vi "Climber.vi"() -> ()   [LabVIEW 2012]
uses:
  ClimberState.ctl
  Robot Global Data.vi
  <vilib>/Rock Robotics/WPI/Relay/WPI_RelayValue.ctl
  <vilib>/Rock Robotics/WPI/Solenoid/WPI_SolenoidSetEnum.vi
  <vilib>/Rock Robotics/WPI/Solenoid/WPI_SolenoidValue.ctl
panel:
  in  "Debug":bool
  in  "Step":T1
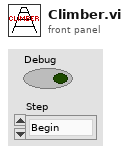
[diagram p1: front panel]
types:
  T1 = typedef "ClimberState.ctl" = enum16{"Begin", "Step 1", "Step 2", "Step 3", "Step 4", "Step 5", "Step 6", "Step 7", "Step 8", "Step 9", "Step 10", "Step 11", "Step 12", "Step 13", "Step 14", "Step 15", "Step 16", "Step 17", "Step 18", "Step 19", "Step 20", "Step 21", "Step 22", "Step 23", "Step 24"}
  T2 = typedef "WPI_RelayValue.ctl" = enum16{"Off", "On", "Forward", "Reverse"}
  T3 = typedef "WPI_SolenoidValue.ctl" = enum16{"Off", "On", "Forward", "Reverse"}
  T4 = typedef "Level state.ctl" = enum16{""}
  T5 = typedef "WPI_RelayDevRef.ctl" = cluster{"DevStatus":errorcluster, "Relay Channel":T6, "Digital Module":T7, "Relay Direction":T8}
  T6 = typedef "FPGA_DIORelayChannel.ctl" = enum8{"Relay 1", "Relay 2", "Relay 3", "Relay 4", "Relay 5", "Relay 6", "Relay 7", "Relay 8", "Invalid"}
  T7 = typedef "FPGA_TypedefDigitalModule.ctl" = enum16{"Digital Module 1", "Digital Module 2"}
  T8 = typedef "WPI_RelayDirection.ctl" = enum16{"Both directions", "Forward only", "Reverse only"}
  T9 = typedef "WPI_MotorControlDeviceRef.ctl" = cluster{"DeviceStatus":errorcluster, "Type":enum16{"PWM", "CAN"}, "PWM":cluster{"Digital Module":T7, "PWM Channel":T10, "DeadBand":T11}, "CAN":cluster{"Device Number":u8, "Control Mode":T12, "Semaphore":T13, "Max Vout":dbl}, "Invert":bool, "TransformRef":T14, "InvTransformRef":T14}
  T10 = typedef "FPGA_DIOPWMChannel.ctl" = enum8{"PWM 1", "PWM 2", "PWM 3", "PWM 4", "PWM 5", "PWM 6", "PWM 7", "PWM 8", "PWM 9", "PWM 10", "Invalid"}
  T11 = typedef "WPI_PWMDeadband.ctl" = cluster{"Name":string, "maxPositivePwm":i32, "minPositivePwm":i32, "centerPwm":i32, "maxNegativePwm":i32, "minNegativePwm":i32, "angularRange":u16}
  T12 = typedef "WPI_CANJaguar_ControlMode.ctl" = enum8{"Percent VBus", "Current", "Speed", "Position", "Voltage"}
  T13 = typedef "Semaphore RefNum" = refnum<k1>
  T14 = typedef "WPI_PWMTransform_ConPane.ctl" = refnum<vi>
  T15 = typedef "WPI_SolenoidDevRef.ctl" = cluster{"DevStatus":errorcluster, "Solenoid Module":T16, "Forward Solenoid Channel":T17, "Reverse Solenoid Channel":T17}
  T16 = typedef "FPGA_TypedefSolenoidModule.ctl" = enum16{"Solenoid Module 1", "Solenoid Module 2"}
  T17 = typedef "WPI_SolenoidChannel.ctl" = enum8{"Solenoid 1", "Solenoid 2", "Solenoid 3", "Solenoid 4", "Solenoid 5", "Solenoid 6", "Solenoid 7", "Solenoid 8", "Invalid"}
  T18 = typedef "WPI_RobotDriveDevRef.ctl" = cluster{"DevStatus":errorcluster, "Motors[]":T9[], "Square Inputs":bool, "Max Output":dbl, "Isochronous":bool}
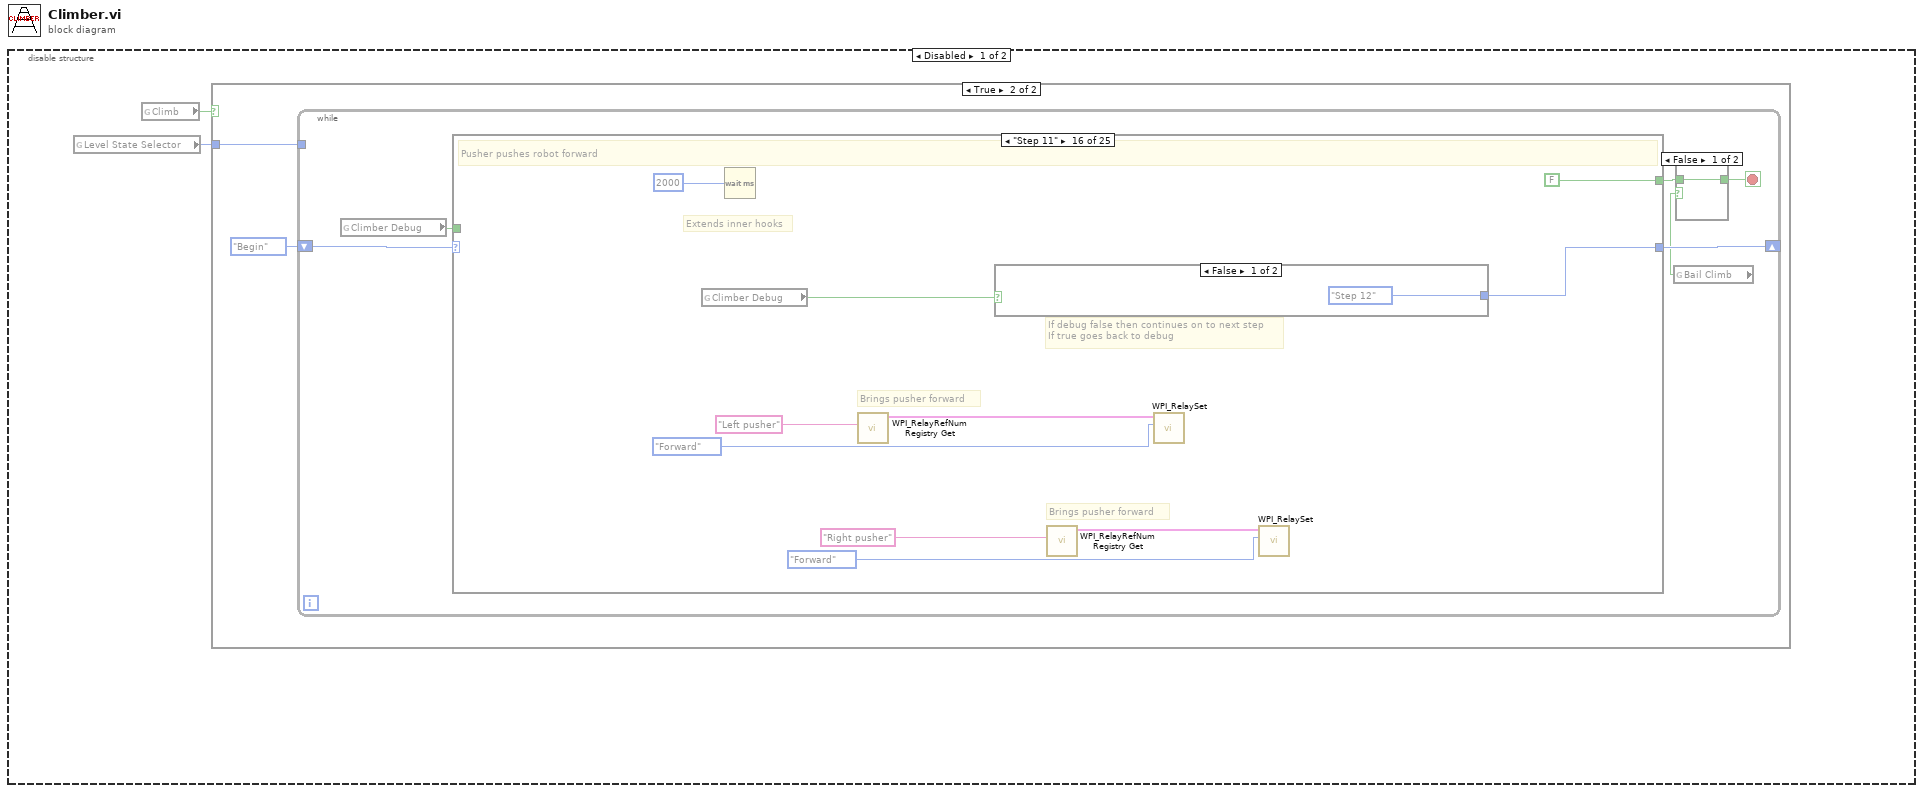
[diagram p0: block diagram]
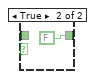
[diagram p3: hidden frame]
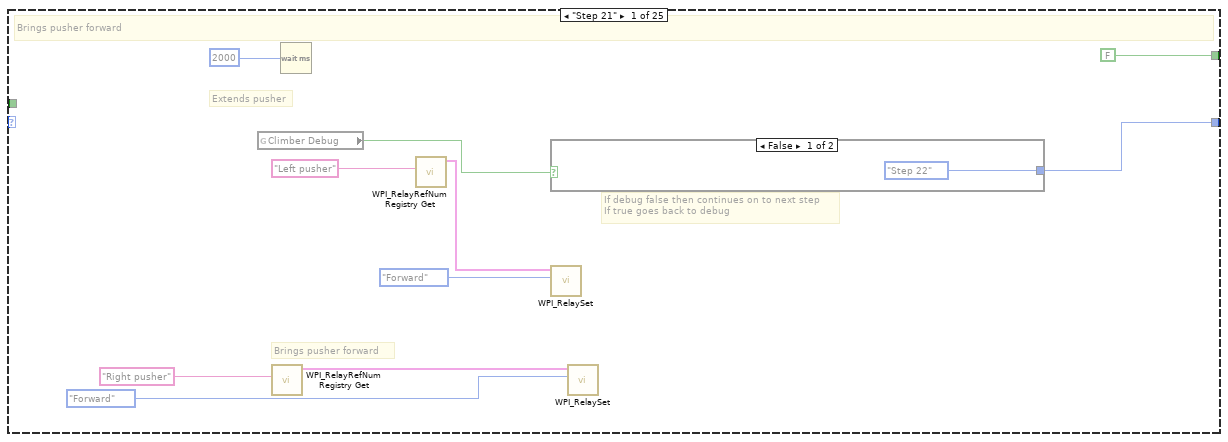
[diagram p4: hidden frame]
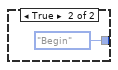
[diagram p5: hidden frame]
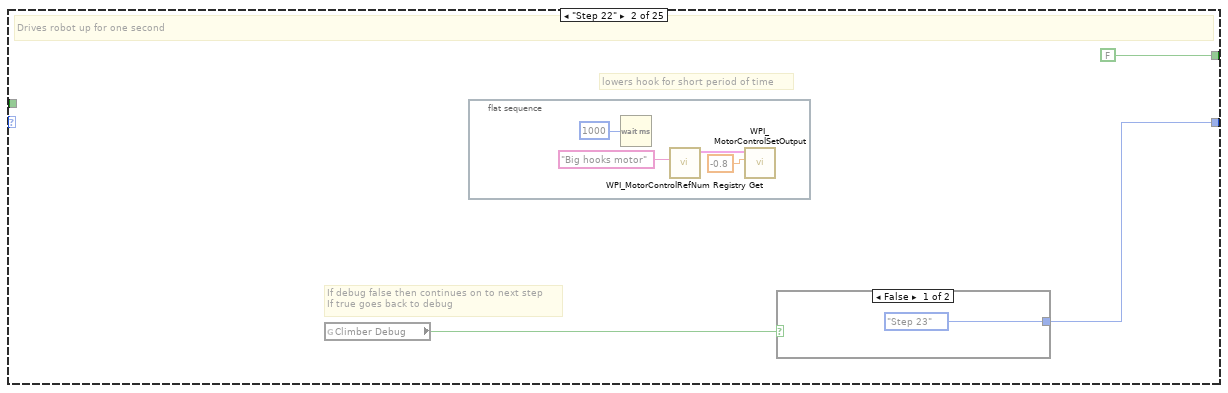
[diagram p6: hidden frame]
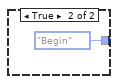
[diagram p7: hidden frame]
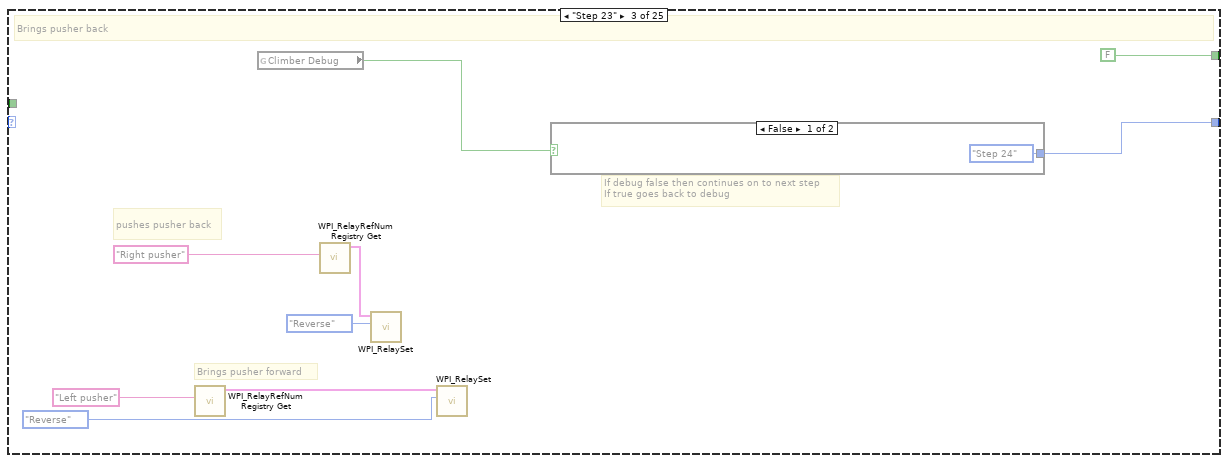
[diagram p8: hidden frame]
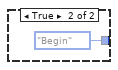
[diagram p9: hidden frame]
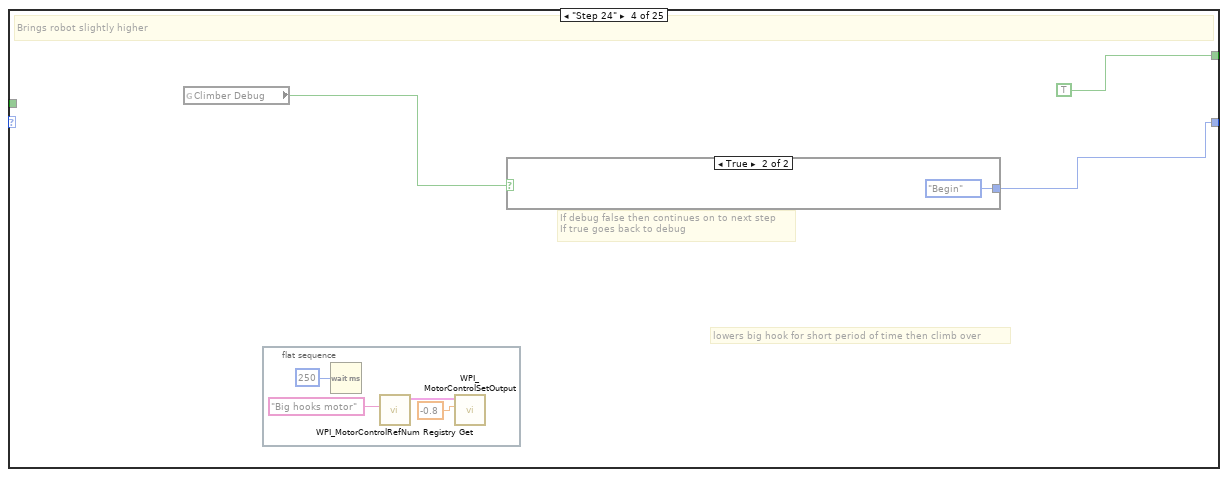
[diagram p10: hidden frame]
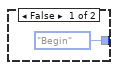
[diagram p11: hidden frame]
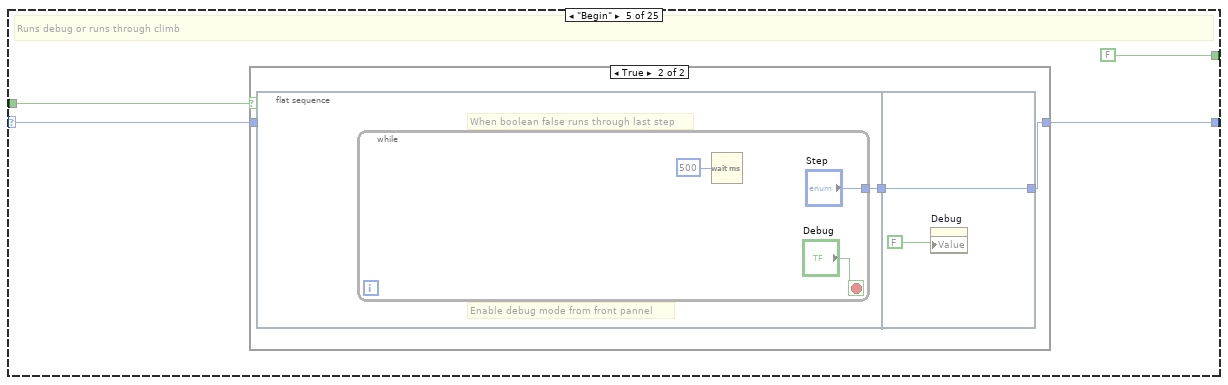
[diagram p12: hidden frame]
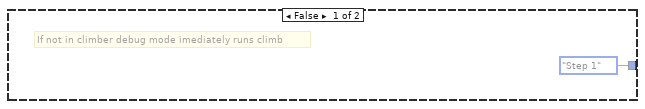
[diagram p13: hidden frame]
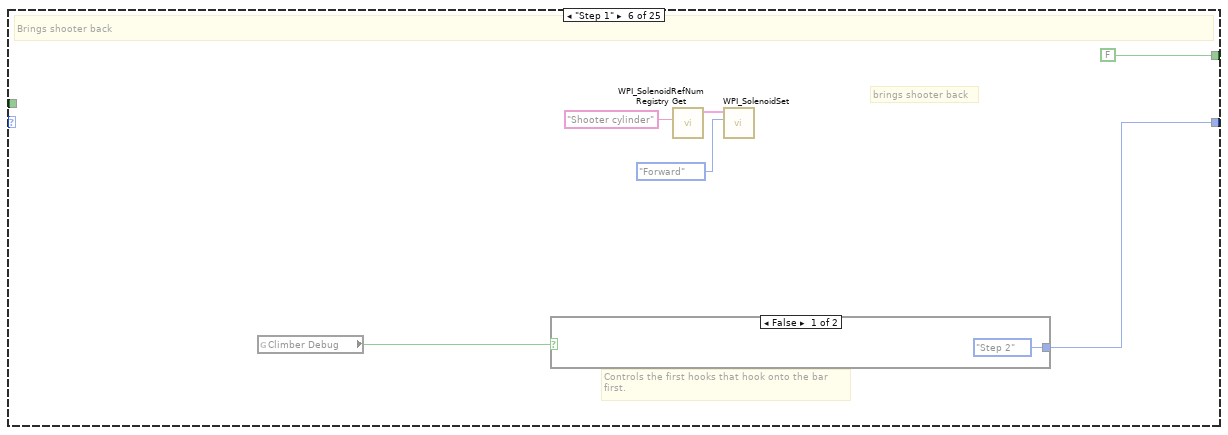
[diagram p14: hidden frame]
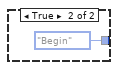
[diagram p15: hidden frame]
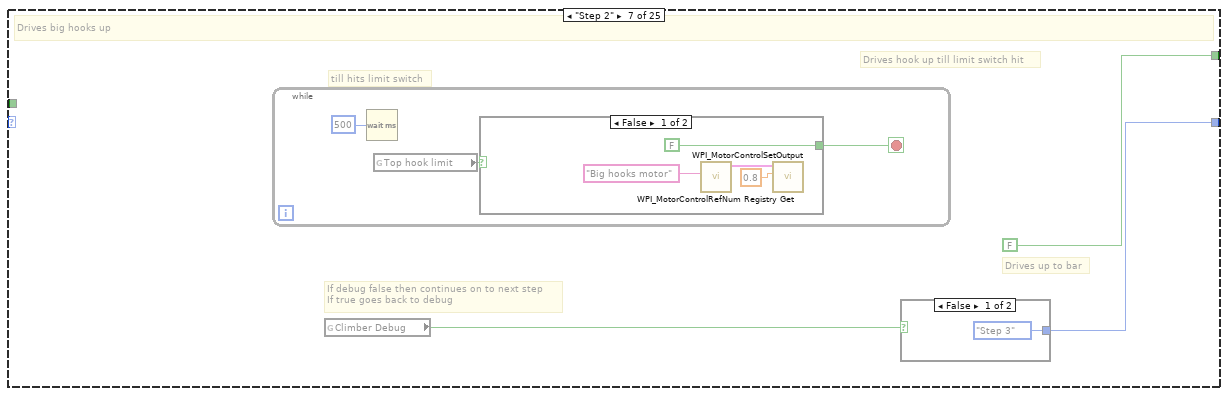
[diagram p16: hidden frame]
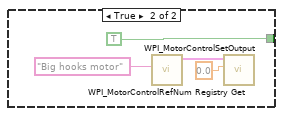
[diagram p17: hidden frame]
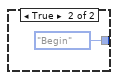
[diagram p18: hidden frame]
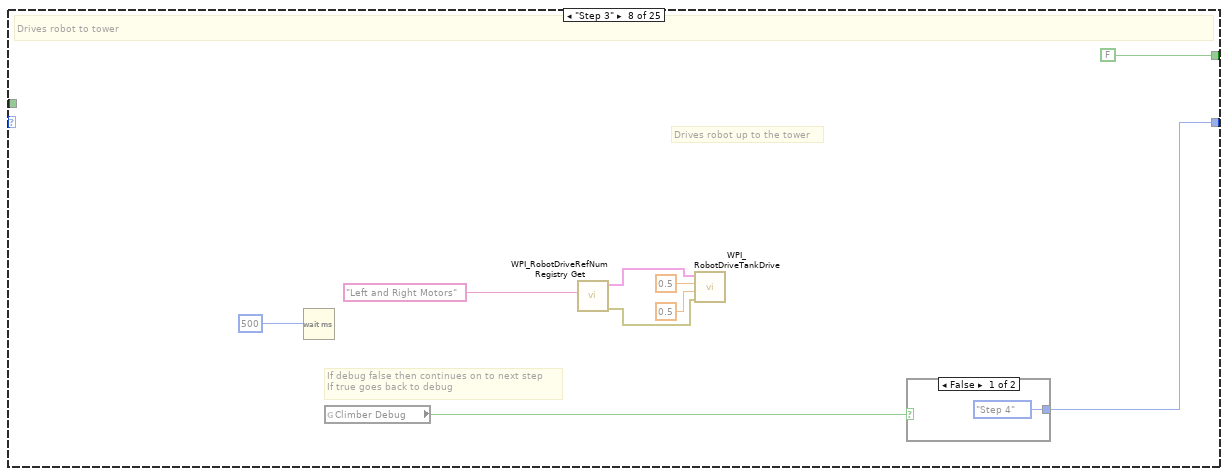
[diagram p19: hidden frame]
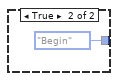
[diagram p20: hidden frame]
diagram:
  n1 = disable-structure shown="Disabled" {
    frame Disabled {
      n2 = global read "Robot Global Data.vi" "Level State Selector"() -> (w2:T4)
      n3 = global read "Robot Global Data.vi" "Climb"() -> (w1:bool)
      n4 = case shown="True" w1 {
        tunnel: w2 -> [_ w3]
        frame False {
        }
        frame True {
          n5 = while {
            shift-right: [w10] -> _
            shift-left: ClimberState."Begin" ("Enum") -> [w9]
            tunnel: w3 -> [_]
            stop <- w7 stop-if-true
            n6 = global read "Robot Global Data.vi" "Climber Debug"() -> (w8:bool)
            n7 = case shown="\"Step 11\"" w9 {
              selector: w9 -> [_ _ _ _ w55 _ _ _ _ _ _ _ _ _ _ _ _ _ _ _ _ _ _ _ _]
              tunnel: [w19 w25 w40 w45 w57 w71 w75 w97 w105 w111 w131 w136 w149 w168 w185 w196 w202 w217 w222 w242 w248 w260 w279 w285 w301] -> w10
              tunnel: [FALSE FALSE FALSE TRUE FALSE FALSE FALSE FALSE FALSE FALSE FALSE FALSE FALSE FALSE FALSE FALSE FALSE FALSE FALSE FALSE FALSE FALSE FALSE FALSE FALSE] -> w6
              tunnel: w8 -> [_ _ _ _ w54 _ _ _ _ _ _ _ _ _ _ _ _ _ _ _ _ _ _ _ _]
              frame "Step 21" {
                # "Brings pusher forward"
                # "If debug false then continues on to next step\nIf true goes back to debug"
                # "Extends pusher"
                # "Brings pusher forward"
                n8 = global read "Robot Global Data.vi" "Climber Debug"() -> (w20:bool)
                n9 = call <vilib>:"WPI_RelayRefNum Registry Get.vi"("refnum name"="Right pusher") -> ("RelayDevRef"=w15:T5)  [unwired: 9 in, 1 out]
                n10 = Wait (ms)(milliseconds to wait=u32 2000) -> ()  [unwired: 1 out]
                n11 = call <vilib>:"WPI_RelayRefNum Registry Get.vi"("refnum name"="Left pusher") -> ("RelayDevRef"=w18:T5)  [unwired: 9 in, 1 out]
                n12 = case shown="False" w20 {
                  tunnel: [ClimberState."Step 22" ("Enum") ClimberState."Begin" ("Enum")] -> w19
                  frame False {
                  }
                  frame True {
                  }
                }
                n13 = call <vilib>:"WPI_RelaySet.vi"("RelayValue"=WPI_RelayValue."Forward", "RelayDevRef"=w18) -> ()  [unwired: 8 in, 2 out]
                n14 = call <vilib>:"WPI_RelaySet.vi"("RelayValue"=WPI_RelayValue."Forward", "RelayDevRef"=w15) -> ()  [unwired: 8 in, 2 out]
              }
              frame "Step 22" {
                # "lowers hook for short period of time"
                # "If debug false then continues on to next step\nIf true goes back to debug"
                # "Drives robot up for one second"
                n15 = global read "Robot Global Data.vi" "Climber Debug"() -> (w26:bool)
                n16 = flat-sequence {
                  frame #0 {
                    n17 = Wait (ms)(milliseconds to wait=u32 1000) -> ()  [unwired: 1 out]
                    n18 = call <vilib>:"WPI_MotorControlRefNum Registry Get.vi"("refnum name"="Big hooks motor") -> ("MotorControlDevRef"=w31:T9)  [unwired: 9 in, 1 out]
                    n19 = call <vilib>:"WPI_MotorControlSetOutput.vi"("Output"=-0.8, "MotorControlDevRef"=w31) -> ()  [unwired: 7 in, 3 out]
                  }
                }
                n20 = case shown="False" w26 {
                  tunnel: [ClimberState."Step 23" ("Enum") ClimberState."Begin" ("Enum")] -> w25
                  frame False {
                  }
                  frame True {
                  }
                }
              }
              frame "Step 23" {
                # "Brings pusher forward"
                # "pushes pusher back"
                # "If debug false then continues on to next step\nIf true goes back to debug"
                # "Brings pusher back"
                n21 = call <vilib>:"WPI_RelayRefNum Registry Get.vi"("refnum name"="Left pusher") -> ("RelayDevRef"=w36:T5)  [unwired: 9 in, 1 out]
                n22 = global read "Robot Global Data.vi" "Climber Debug"() -> (w41:bool)
                n23 = call <vilib>:"WPI_RelayRefNum Registry Get.vi"("refnum name"="Right pusher") -> ("RelayDevRef"=w39:T5)  [unwired: 9 in, 1 out]
                n24 = call <vilib>:"WPI_RelaySet.vi"("RelayValue"=WPI_RelayValue."Reverse", "RelayDevRef"=w39) -> ()  [unwired: 8 in, 2 out]
                n25 = call <vilib>:"WPI_RelaySet.vi"("RelayValue"=WPI_RelayValue."Reverse", "RelayDevRef"=w36) -> ()  [unwired: 8 in, 2 out]
                n26 = case shown="False" w41 {
                  tunnel: [ClimberState."Step 24" ("Enum") ClimberState."Begin" ("Enum")] -> w40
                  frame False {
                  }
                  frame True {
                  }
                }
              }
              frame "Step 24" {
                # "lowers big hook for short period of time then climb over"
                # "If debug false then continues on to next step\nIf true goes back to debug"
                # "Brings robot slightly higher"
                n27 = global read "Robot Global Data.vi" "Climber Debug"() -> (w47:bool)
                n28 = flat-sequence {
                  frame #0 {
                    n29 = Wait (ms)(milliseconds to wait=u32 250) -> ()  [unwired: 1 out]
                    n30 = call <vilib>:"WPI_MotorControlRefNum Registry Get.vi"("refnum name"="Big hooks motor") -> ("MotorControlDevRef"=w51:T9)  [unwired: 9 in, 1 out]
                    n31 = call <vilib>:"WPI_MotorControlSetOutput.vi"("Output"=-0.8, "MotorControlDevRef"=w51) -> ()  [unwired: 7 in, 3 out]
                  }
                }
                n32 = case shown="True" w47 {
                  tunnel: [ClimberState."Begin" ("Enum") ClimberState."Begin" ("Enum")] -> w45
                  frame False {
                  }
                  frame True {
                  }
                }
              }
              frame "Begin" {
                # "Runs debug or runs through climb"
                n33 = case shown="True" w54 {
                  tunnel: [ClimberState."Step 1" ("Enum") w60] -> w57
                  tunnel: w55 -> [_ _]
                  frame False {
                    # "If not in climber debug mode imediately runs climb"
                  }
                  frame True {
                    n34 = flat-sequence {
                      tunnel: [w61] -> w59
                      tunnel: [w66] -> w60
                      tunnel: w59 -> [w66]
                      frame #0 {
                        # "When boolean false runs through last step"
                        # "Enable debug mode from front pannel"
                        n35 = while {
                          tunnel: ["Step"] -> w61
                          stop <- "Debug" stop-if-true
                          n36 = Wait (ms)(milliseconds to wait=u32 500) -> ()  [unwired: 1 out]
                        }
                      }
                      frame #1 {
                        n37 = property on="Debug" class="Bool (strict)"("Value"=FALSE ("Debug")) -> ()  [unwired: 2 in, 2 out]
                      }
                    }
                  }
                }
              }
              frame "Step 1" {
                # "brings shooter back"
                # "Controls the first hooks that hook onto the bar\nfirst."
                # "Brings shooter back"
                n38 = global read "Robot Global Data.vi" "Climber Debug"() -> (w70:bool)
                n39 = case shown="False" w70 {
                  tunnel: [ClimberState."Step 2" ("Enum") ClimberState."Begin" ("Enum")] -> w71
                  frame False {
                  }
                  frame True {
                  }
                }
                n40 = call <vilib>:"WPI_SolenoidRefNum Registry Get.vi"("refnum name"="Shooter cylinder") -> ("SolenoidDevRef"=w68:T15)  [unwired: 9 in, 1 out]
                n41 = call-poly <vilib>:"WPI_SolenoidSet.vi"("Value"=WPI_SolenoidValue."Forward", "SolenoidDevRef"=w68) -> ()  [unwired: 8 in, 2 out]
              }
              frame "Step 2" {
                # "Drives hook up till limit switch hit"
                # "till hits limit switch"
                # "If debug false then continues on to next step\nIf true goes back to debug"
                # "Drives up to bar"
                # "Drives big hooks up"
                n42 = while {
                  stop <- w80 stop-if-true
                  n43 = Wait (ms)(milliseconds to wait=u32 500) -> ()  [unwired: 1 out]
                  n44 = global read "Robot Global Data.vi" "Top hook limit"() -> (w78:bool)
                  n45 = case shown="False" w78 {
                    tunnel: [FALSE TRUE] -> w80
                    frame False {
                      n46 = call <vilib>:"WPI_MotorControlRefNum Registry Get.vi"("refnum name"="Big hooks motor") -> ("MotorControlDevRef"=w82:T9)  [unwired: 9 in, 1 out]
                      n47 = call <vilib>:"WPI_MotorControlSetOutput.vi"("Output"=0.8, "MotorControlDevRef"=w82) -> ()  [unwired: 7 in, 3 out]
                    }
                    frame True {
                      n48 = call <vilib>:"WPI_MotorControlRefNum Registry Get.vi"("refnum name"="Big hooks motor") -> ("MotorControlDevRef"=w88:T9)  [unwired: 9 in, 1 out]
                      n49 = call <vilib>:"WPI_MotorControlSetOutput.vi"("Output"=0.0, "MotorControlDevRef"=w88) -> ()  [unwired: 7 in, 3 out]
                    }
                  }
                }
                n50 = global read "Robot Global Data.vi" "Climber Debug"() -> (w76:bool)
                n51 = case shown="False" w76 {
                  tunnel: [ClimberState."Step 3" ("Enum") ClimberState."Begin" ("Enum")] -> w75
                  frame False {
                  }
                  frame True {
                  }
                }
              }
              frame "Step 3" {
                # "Drives robot up to the tower"
                # "If debug false then continues on to next step\nIf true goes back to debug"
                # "Drives robot to tower"
                n52 = Wait (ms)(milliseconds to wait=u32 500) -> ()  [unwired: 1 out]
                n53 = global read "Robot Global Data.vi" "Climber Debug"() -> (w98:bool)
                n54 = call <vilib>:"WPI_RobotDriveRefNum Registry Get.vi"("refnum name"="Left and Right Motors") -> ("error out"=w96:errorcluster, "RobotDriveDevRef"=w95:T18)  [unwired: 1 in, 8 out]
                n55 = call <vilib>:"WPI_RobotDriveTankDrive.vi"("error in (no error)"=w96, "Right axis value"=0.5, "Left axis value"=0.5, "RobotDriveDevRef"=w95) -> ()  [unwired: 5 in, 3 out]
                n56 = case shown="False" w98 {
                  tunnel: [ClimberState."Step 4" ("Enum") ClimberState."Begin" ("Enum")] -> w97
                  frame False {
                  }
                  frame True {
                  }
                }
              }
              frame "Step 4" {
                # "Makes sure that Ratchet is engaged"
                # "If debug false then continues on to next step\nIf true goes back to debug"
                # "Brings Ratchet Forward to Ensure that it is Engaged"
                n57 = global read "Robot Global Data.vi" "Climber Debug"() -> (w106:bool)
                n58 = case shown="False" w106 {
                  tunnel: [ClimberState."Step 5" ("Enum") ClimberState."Begin" ("Enum")] -> w105
                  frame False {
                  }
                  frame True {
                  }
                }
                n59 = call <vilib>:"WPI_SolenoidRefNum Registry Get.vi"("refnum name"="Big hooks lock") -> ("SolenoidDevRef"=w103:T15)  [unwired: 9 in, 1 out]
                n60 = call-poly <vilib>:"WPI_SolenoidSet.vi"("Value"=WPI_SolenoidValue."Forward", "SolenoidDevRef"=w103) -> ()  [unwired: 8 in, 2 out]
                n61 = Wait (ms)(milliseconds to wait=u32 2000 ("millisecond timer value")) -> ()  [unwired: 1 out]
              }
              frame "Step 5" {
                # "Drives big hook down until limit switch hit"
                # "If debug false then continues on to next step\nIf true goes back to debug"
                # "Drives Big Hooks Down Until Limit Switch Hit"
                n62 = global read "Robot Global Data.vi" "Climber Debug"() -> (w112:bool)
                n63 = while {
                  stop <- w116 stop-if-true
                  n64 = Wait (ms)(milliseconds to wait=u32 500) -> ()  [unwired: 1 out]
                  n65 = global read "Robot Global Data.vi" "Top hook limit"() -> (w114:bool)
                  n66 = case shown="True" w114 {
                    tunnel: [TRUE FALSE] -> w116
                    frame False {
                      n67 = call <vilib>:"WPI_MotorControlRefNum Registry Get.vi"("refnum name"="Big hook") -> ("MotorControlDevRef"=w118:T9)  [unwired: 9 in, 1 out]
                      n68 = call <vilib>:"WPI_MotorControlSetOutput.vi"("Output"=0.0, "MotorControlDevRef"=w118) -> ()  [unwired: 7 in, 3 out]
                    }
                    frame True {
                      n69 = call <vilib>:"WPI_MotorControlRefNum Registry Get.vi"("refnum name"="Big hook motor") -> ("MotorControlDevRef"=w124:T9)  [unwired: 9 in, 1 out]
                      n70 = call <vilib>:"WPI_MotorControlSetOutput.vi"("Output"=-0.8, "MotorControlDevRef"=w124) -> ()  [unwired: 7 in, 3 out]
                    }
                  }
                }
                n71 = case shown="False" w112 {
                  tunnel: [ClimberState."Step 6" ("Enum") ClimberState."Begin" ("Enum")] -> w111
                  frame False {
                  }
                  frame True {
                  }
                }
              }
              frame "Step 6" {
                # "pushes inner hooks forward"
                # "Extends Outer Hook"
                # "If debug false then continues on to next step\nIf true goes back to debug"
                # "Brings Small Hooks Forward onto Bar"
                n72 = global read "Robot Global Data.vi" "Climber Debug"() -> (w132:bool)
                n73 = call <vilib>:"WPI_RelayRefNum Registry Get.vi"("refnum name"="Small hooks") -> ("RelayDevRef"=w130:T5)  [unwired: 9 in, 1 out]
                n74 = call <vilib>:"WPI_RelaySet.vi"("RelayValue"=WPI_RelayValue."Forward", "RelayDevRef"=w130) -> ()  [unwired: 8 in, 2 out]
                n75 = Wait (ms)(milliseconds to wait=u32 1000) -> ()  [unwired: 1 out]
                n76 = case shown="False" w132 {
                  tunnel: [ClimberState."Step 7" ("Enum") ClimberState."Begin" ("Enum")] -> w131
                  frame False {
                  }
                  frame True {
                  }
                }
              }
              frame "Step 7" {
                # "Brings ratchet back then drives down for short moment"
                # "If debug false then continues on to next step\nIf true goes back to debug"
                # "Brings ratchet back and drives down"
                n77 = Wait (ms)(milliseconds to wait=u32 2000 ("millisecond timer value")) -> ()  [unwired: 1 out]
                n78 = global read "Robot Global Data.vi" "Climber Debug"() -> (w137:bool)
                n79 = flat-sequence {
                  frame #0 {
                    n80 = call <vilib>:"WPI_SolenoidRefNum Registry Get.vi"("refnum name"="Big hooks lock") -> ("SolenoidDevRef"=w141:T15)  [unwired: 9 in, 1 out]
                    n81 = call-poly <vilib>:"WPI_SolenoidSet.vi"("Value"=WPI_SolenoidValue."Reverse", "SolenoidDevRef"=w141) -> ()  [unwired: 8 in, 2 out]
                  }
                  frame #1 {
                    n82 = call <vilib>:"WPI_MotorControlRefNum Registry Get.vi"("refnum name"="Big hooks motor") -> ("MotorControlDevRef"=w146:T9)  [unwired: 9 in, 1 out]
                    n83 = Wait (ms)(milliseconds to wait=u32 250) -> ()  [unwired: 1 out]
                    n84 = call <vilib>:"WPI_MotorControlSetOutput.vi"("Output"=-0.8, "MotorControlDevRef"=w146) -> ()  [unwired: 7 in, 3 out]
                  }
                }
                n85 = case shown="False" w137 {
                  tunnel: [ClimberState."Step 8" ("Enum") ClimberState."Begin" ("Enum")] -> w136
                  frame False {
                  }
                  frame True {
                  }
                }
              }
              frame "Step 8" {
                # "till hits limit switch"
                # "If debug false then continues on to next step\nIf true goes back to debug"
                # "Extends inner hooks"
                # "Brings big hook up until limit switch hit"
                n86 = global read "Robot Global Data.vi" "Climber Debug"() -> (w150:bool)
                n87 = while {
                  stop <- w154 stop-if-true
                  n88 = Wait (ms)(milliseconds to wait=u32 500) -> ()  [unwired: 1 out]
                  n89 = global read "Robot Global Data.vi" "Top hook limit"() -> (w153:bool)
                  n90 = case shown="False" w153 {
                    tunnel: [FALSE TRUE] -> w154
                    frame False {
                      n91 = call <vilib>:"WPI_MotorControlRefNum Registry Get.vi"("refnum name"="Big hooks motor") -> ("MotorControlDevRef"=w156:T9)  [unwired: 9 in, 1 out]
                      n92 = call <vilib>:"WPI_MotorControlSetOutput.vi"("Output"=0.8, "MotorControlDevRef"=w156) -> ()  [unwired: 7 in, 3 out]
                    }
                    frame True {
                      n93 = call <vilib>:"WPI_MotorControlRefNum Registry Get.vi"("refnum name"="Big hooks motor") -> ("MotorControlDevRef"=w162:T9)  [unwired: 9 in, 1 out]
                      n94 = call <vilib>:"WPI_MotorControlSetOutput.vi"("Output"=0.0, "MotorControlDevRef"=w162) -> ()  [unwired: 7 in, 3 out]
                    }
                  }
                }
                n95 = case shown="False" w150 {
                  tunnel: [ClimberState."Step 9" ("Enum") ClimberState."Begin" ("Enum")] -> w149
                  frame False {
                  }
                  frame True {
                  }
                }
              }
              frame "Step 9" {
                # "If debug false then continues on to next step\nIf true goes back to debug"
                # "pushes pusher forward"
                # "Extends inner hooks"
                # "Brings Ratchet forward and lowers big hook"
                n96 = call <vilib>:"WPI_SolenoidRefNum Registry Get.vi"("refnum name"="Big hooks lock") -> ("SolenoidDevRef"=w166:T15)  [unwired: 9 in, 1 out]
                n97 = call-poly <vilib>:"WPI_SolenoidSet.vi"("Value"=WPI_SolenoidValue."Forward", "SolenoidDevRef"=w166) -> ()  [unwired: 8 in, 2 out]
                n98 = global read "Robot Global Data.vi" "Climber Debug"() -> (w169:bool)
                n99 = Wait (ms)(milliseconds to wait=u32 2000) -> ()  [unwired: 1 out]
                n100 = while {
                  stop <- w173 stop-if-true
                  n101 = global read "Robot Global Data.vi" "Big Hooks on Bar"() -> (w174:bool)
                  n102 = Wait (ms)(milliseconds to wait=u32 1000) -> ()  [unwired: 1 out]
                  n103 = case shown="False" w174 {
                    tunnel: [FALSE TRUE] -> w173
                    frame False {
                      # "Lowers the big hook"
                      n104 = call <vilib>:"WPI_MotorControlRefNum Registry Get.vi"("refnum name"="Big hooks motor") -> ("MotorControlDevRef"=w178:T9)  [unwired: 9 in, 1 out]
                      n105 = call <vilib>:"WPI_MotorControlSetOutput.vi"("Output"=-0.8, "MotorControlDevRef"=w178) -> ()  [unwired: 7 in, 3 out]
                    }
                    frame True {
                    }
                  }
                }
                n106 = case shown="False" w169 {
                  tunnel: [ClimberState."Step 10" ("Enum") ClimberState."Begin" ("Enum")] -> w168
                  frame False {
                  }
                  frame True {
                  }
                }
              }
              frame "Step 10" {
                # "Bring small inner hooks back"
                # "If debug false then continues on to next step\nIf true goes back to debug"
                # "Brings small inner hooks back"
                n107 = global read "Robot Global Data.vi" "Climber Debug"() -> (w186:bool)
                n108 = call <vilib>:"WPI_RelayRefNum Registry Get.vi"("refnum name"="Small hooks") -> ("RelayDevRef"=w184:T5)  [unwired: 9 in, 1 out]
                n109 = case shown="False" w186 {
                  tunnel: [ClimberState."Step 11" ("Enum") ClimberState."Begin" ("Enum")] -> w185
                  frame False {
                  }
                  frame True {
                  }
                }
                n110 = call <vilib>:"WPI_RelaySet.vi"("RelayValue"=WPI_RelayValue."Reverse", "RelayDevRef"=w184) -> ()  [unwired: 8 in, 2 out]
              }
              frame "Step 11" {
                # "Brings pusher forward"
                # "If debug false then continues on to next step\nIf true goes back to debug"
                # "Brings pusher forward"
                # "Extends inner hooks"
                # "Pusher pushes robot forward"
                n111 = global read "Robot Global Data.vi" "Climber Debug"() -> (w197:bool)
                n112 = Wait (ms)(milliseconds to wait=u32 2000) -> ()  [unwired: 1 out]
                n113 = call <vilib>:"WPI_RelayRefNum Registry Get.vi"("refnum name"="Left pusher") -> ("RelayDevRef"=w195:T5)  [unwired: 9 in, 1 out]
                n114 = case shown="False" w197 {
                  tunnel: [ClimberState."Step 12" ("Enum") ClimberState."Begin" ("Enum")] -> w196
                  frame False {
                  }
                  frame True {
                  }
                }
                n115 = call <vilib>:"WPI_RelayRefNum Registry Get.vi"("refnum name"="Right pusher") -> ("RelayDevRef"=w192:T5)  [unwired: 9 in, 1 out]
                n116 = call <vilib>:"WPI_RelaySet.vi"("RelayValue"=WPI_RelayValue."Forward", "RelayDevRef"=w195) -> ()  [unwired: 8 in, 2 out]
                n117 = call <vilib>:"WPI_RelaySet.vi"("RelayValue"=WPI_RelayValue."Forward", "RelayDevRef"=w192) -> ()  [unwired: 8 in, 2 out]
              }
              frame "Step 12" {
                # "lowers big hook for short period of time"
                # "If debug false then continues on to next step\nIf true goes back to debug"
                # "Extends Outer Hook"
                # "Robot lowers for one second"
                n118 = global read "Robot Global Data.vi" "Climber Debug"() -> (w203:bool)
                n119 = flat-sequence {
                  frame #0 {
                    n120 = Wait (ms)(milliseconds to wait=u32 1000) -> ()  [unwired: 1 out]
                    n121 = call <vilib>:"WPI_MotorControlRefNum Registry Get.vi"("refnum name"="Big hooks motor") -> ("MotorControlDevRef"=w208:T9)  [unwired: 9 in, 1 out]
                    n122 = call <vilib>:"WPI_MotorControlSetOutput.vi"("Output"=-0.8, "MotorControlDevRef"=w208) -> ()  [unwired: 7 in, 3 out]
                  }
                }
                n123 = case shown="False" w203 {
                  tunnel: [ClimberState."Step 13" ("Enum") ClimberState."Begin" ("Enum")] -> w202
                  frame False {
                  }
                  frame True {
                  }
                }
              }
              frame "Step 13" {
                # "brings pusher cyliner back"
                # "If debug false then continues on to next step\nIf true goes back to debug"
                # "Pusher reverses"
                n124 = global read "Robot Global Data.vi" "Climber Debug"() -> (w218:bool)
                n125 = call <vilib>:"WPI_RelayRefNum Registry Get.vi"("refnum name"="Right pusher") -> ("RelayDevRef"=w213:T5)  [unwired: 9 in, 1 out]
                n126 = call <vilib>:"WPI_RelayRefNum Registry Get.vi"("refnum name"="Left pusher") -> ("RelayDevRef"=w216:T5)  [unwired: 9 in, 1 out]
                n127 = call <vilib>:"WPI_RelaySet.vi"("RelayValue"=WPI_RelayValue."Reverse", "RelayDevRef"=w213) -> ()  [unwired: 8 in, 2 out]
                n128 = case shown="False" w218 {
                  tunnel: [ClimberState."Step 14" ("Enum") ClimberState."Begin" ("Enum")] -> w217
                  frame False {
                  }
                  frame True {
                  }
                }
                n129 = call <vilib>:"WPI_RelaySet.vi"("RelayValue"=WPI_RelayValue."Reverse", "RelayDevRef"=w216) -> ()  [unwired: 8 in, 2 out]
              }
              frame "Step 14" {
                # "till hits limit switch"
                # "lowers big hook"
                # "Robot lowers itself rest of way down"
                n130 = global read "Robot Global Data.vi" "Climber Debug"() -> (w223:bool)
                n131 = while {
                  stop <- w228 stop-if-true
                  n132 = global read "Robot Global Data.vi" "Lower hook limit"() -> (w226:bool)
                  n133 = Wait (ms)(milliseconds to wait=u32 500) -> ()  [unwired: 1 out]
                  n134 = case shown="False" w226 {
                    tunnel: [FALSE TRUE] -> w228
                    frame False {
                      n135 = call <vilib>:"WPI_MotorControlRefNum Registry Get.vi"("refnum name"="Big hooks motor") -> ("MotorControlDevRef"=w230:T9)  [unwired: 9 in, 1 out]
                      n136 = call <vilib>:"WPI_MotorControlSetOutput.vi"("Output"=-0.8, "MotorControlDevRef"=w230) -> ()  [unwired: 7 in, 3 out]
                    }
                    frame True {
                      n137 = call <vilib>:"WPI_MotorControlRefNum Registry Get.vi"("refnum name"="Big hook") -> ("MotorControlDevRef"=w236:T9)  [unwired: 9 in, 1 out]
                      n138 = call <vilib>:"WPI_MotorControlSetOutput.vi"("Output"=0.0, "MotorControlDevRef"=w236) -> ()  [unwired: 7 in, 3 out]
                    }
                  }
                }
                n139 = case shown="False" w223 {
                  tunnel: [ClimberState."Step 15" ("Enum") ClimberState."Begin" ("Enum")] -> w222
                  frame False {
                  }
                  frame True {
                  }
                }
                n140 = Wait (ms)(milliseconds to wait=u32 2000 ("millisecond timer value")) -> ()  [unwired: 1 out]
              }
              frame "Step 15" {
                # "brings small inner hooks forward"
                # "If debug false then continues on to next step\nIf true goes back to debug"
                # "Brings small hooks forward till they are on bar"
                n141 = global read "Robot Global Data.vi" "Climber Debug"() -> (w243:bool)
                n142 = Wait (ms)(milliseconds to wait=u32 2000) -> ()  [unwired: 1 out]
                n143 = call <vilib>:"WPI_RelayRefNum Registry Get.vi"("refnum name"="Small hooks") -> ("RelayDevRef"=w241:T5)  [unwired: 9 in, 1 out]
                n144 = case shown="False" w243 {
                  tunnel: [ClimberState."Step 16" ("Enum") ClimberState."Begin" ("Enum")] -> w242
                  frame False {
                  }
                  frame True {
                  }
                }
                n145 = call <vilib>:"WPI_RelaySet.vi"("RelayValue"=WPI_RelayValue."Forward", "RelayDevRef"=w241) -> ()  [unwired: 8 in, 2 out]
              }
              frame "Step 16" {
                # "brings ratchet back and then brings big hook down"
                # "If debug false then continues on to next step\nIf true goes back to debug"
                # "Brings ratchet back and drives down"
                n146 = flat-sequence {
                  frame #0 {
                    n147 = call <vilib>:"WPI_SolenoidRefNum Registry Get.vi"("refnum name"="Big hooks lock") -> ("SolenoidDevRef"=w252:T15)  [unwired: 9 in, 1 out]
                    n148 = call-poly <vilib>:"WPI_SolenoidSet.vi"("Value"=WPI_SolenoidValue."Reverse", "SolenoidDevRef"=w252) -> ()  [unwired: 8 in, 2 out]
                  }
                  frame #1 {
                    n149 = call <vilib>:"WPI_MotorControlRefNum Registry Get.vi"("refnum name"="Big hooks motor") -> ("MotorControlDevRef"=w257:T9)  [unwired: 9 in, 1 out]
                    n150 = Wait (ms)(milliseconds to wait=u32 500) -> ()  [unwired: 1 out]
                    n151 = call <vilib>:"WPI_MotorControlSetOutput.vi"("Output"=-0.8, "MotorControlDevRef"=w257) -> ()  [unwired: 7 in, 3 out]
                  }
                }
                n152 = global read "Robot Global Data.vi" "Climber Debug"() -> (w249:bool)
                n153 = case shown="False" w249 {
                  tunnel: [ClimberState."Step 17" ("Enum") ClimberState."Begin" ("Enum")] -> w248
                  frame False {
                  }
                  frame True {
                  }
                }
              }
              frame "Step 17" {
                # "brings big hook up"
                # "till hits limit switch"
                # "Brings big hook up until limit switch activated"
                n154 = while {
                  stop <- w265 stop-if-true
                  n155 = Wait (ms)(milliseconds to wait=u32 500) -> ()  [unwired: 1 out]
                  n156 = global read "Robot Global Data.vi" "Top hook limit"() -> (w263:bool)
                  n157 = case shown="False" w263 {
                    tunnel: [FALSE TRUE] -> w265
                    frame False {
                      n158 = call <vilib>:"WPI_MotorControlRefNum Registry Get.vi"("refnum name"="Big hooks motor") -> ("MotorControlDevRef"=w267:T9)  [unwired: 9 in, 1 out]
                      n159 = call <vilib>:"WPI_MotorControlSetOutput.vi"("Output"=0.8, "MotorControlDevRef"=w267) -> ()  [unwired: 7 in, 3 out]
                    }
                    frame True {
                      n160 = call <vilib>:"WPI_MotorControlRefNum Registry Get.vi"("refnum name"="Big hook") -> ("MotorControlDevRef"=w273:T9)  [unwired: 9 in, 1 out]
                      n161 = call <vilib>:"WPI_MotorControlSetOutput.vi"("Output"=0.0, "MotorControlDevRef"=w273) -> ()  [unwired: 7 in, 3 out]
                    }
                  }
                }
                n162 = global read "Robot Global Data.vi" "Climber Debug"() -> (w261:bool)
                n163 = case shown="False" w261 {
                  tunnel: [ClimberState."Step 18" ("Enum") ClimberState."Begin" ("Enum")] -> w260
                  frame False {
                  }
                  frame True {
                  }
                }
              }
              frame "Step 18" {
                # "engage ratchet"
                # "If debug false then continues on to next step\nIf true goes back to debug"
                # "Extends inner hooks"
                # "Brings ratchet forward"
                n164 = global read "Robot Global Data.vi" "Climber Debug"() -> (w280:bool)
                n165 = Wait (ms)(milliseconds to wait=u32 2000) -> ()  [unwired: 1 out]
                n166 = call <vilib>:"WPI_SolenoidRefNum Registry Get.vi"("refnum name"="Big hooks lock") -> ("SolenoidDevRef"=w277:T15)  [unwired: 9 in, 1 out]
                n167 = call-poly <vilib>:"WPI_SolenoidSet.vi"("Value"=WPI_SolenoidValue."Forward", "SolenoidDevRef"=w277) -> ()  [unwired: 8 in, 2 out]
                n168 = case shown="False" w280 {
                  tunnel: [ClimberState."Step 19" ("Enum") ClimberState."Begin" ("Enum")] -> w279
                  frame False {
                  }
                  frame True {
                  }
                }
              }
              frame "Step 19" {
                # "If debug false then continues on to next step\nIf true goes back to debug"
                # "Brings big hooks down until they are on bar"
                n169 = while {
                  stop <- w289 stop-if-true
                  n170 = global read "Robot Global Data.vi" "Big Hooks on Bar"() -> (w290:bool)
                  n171 = Wait (ms)(milliseconds to wait=u32 500) -> ()  [unwired: 1 out]
                  n172 = case shown="False" w290 {
                    tunnel: [FALSE TRUE] -> w289
                    frame False {
                      # "Lowers the big hook until proximity hit"
                      n173 = call <vilib>:"WPI_MotorControlRefNum Registry Get.vi"("refnum name"="Big hooks motor") -> ("MotorControlDevRef"=w294:T9)  [unwired: 9 in, 1 out]
                      n174 = call <vilib>:"WPI_MotorControlSetOutput.vi"("Output"=-0.8, "MotorControlDevRef"=w294) -> ()  [unwired: 7 in, 3 out]
                    }
                    frame True {
                    }
                  }
                }
                n175 = global read "Robot Global Data.vi" "Climber Debug"() -> (w286:bool)
                n176 = case shown="False" w286 {
                  tunnel: [ClimberState."Step 20" ("Enum") ClimberState."Begin" ("Enum")] -> w285
                  frame False {
                  }
                  frame True {
                  }
                }
              }
              frame "Step 20" {
                # "disengage small hooks"
                # "If debug false then continues on to next step\nIf true goes back to debug"
                # "Brings small hooks back"
                n177 = global read "Robot Global Data.vi" "Climber Debug"() -> (w302:bool)
                n178 = call <vilib>:"WPI_RelayRefNum Registry Get.vi"("refnum name"="Small hooks") -> ("RelayDevRef"=w300:T5)  [unwired: 9 in, 1 out]
                n179 = case shown="False" w302 {
                  tunnel: [ClimberState."Step 21" ("Enum") ClimberState."Begin" ("Enum")] -> w301
                  frame False {
                  }
                  frame True {
                  }
                }
                n180 = call <vilib>:"WPI_RelaySet.vi"("RelayValue"=WPI_RelayValue."Reverse", "RelayDevRef"=w300) -> ()  [unwired: 8 in, 2 out]
                n181 = Wait (ms)(milliseconds to wait=u32 2000 ("millisecond timer value")) -> ()  [unwired: 1 out]
              }
            }
            n182 = global read "Robot Global Data.vi" "Bail Climb"() -> (w5:bool)
            n183 = case shown="False" w5 {
              tunnel: [w11 FALSE] -> w7
              tunnel: w6 -> [w11 _]
              frame False {
              }
              frame True {
              }
            }
          }
        }
      }
    }
    frame Enabled {
    }
  }
